vi "Interpolate Points_new.vi"(1 "End Point":cluster{"X":dbl, "Y":dbl}, 2 "Points number":dbl, 3 "Start Point":cluster{"X":dbl, "Y":dbl}) -> (0 "Output Point Array":cluster{"X":dbl, "Y":dbl}[](array[cluster]))   [LabVIEW 2013]
doc: "This VI interpolates at specified intervals between two points."
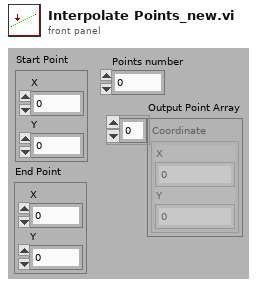
[diagram p1: front panel]
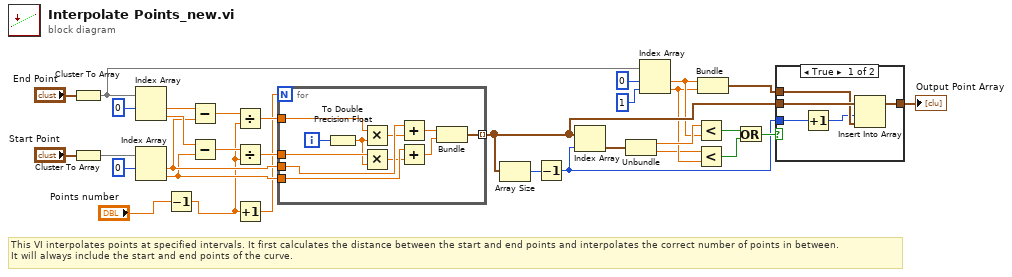
[diagram p0: block diagram]
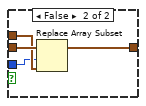
[diagram p2: hidden frame]
diagram:
  # "This VI interpolates points at specified intervals. It first calculates the distance between the start and end points and interpolates the correct number of points in between. \nIt will always include the start and end points of the curve."
  n1 = Cluster To Array(cluster="End Point") -> (array=w15:dbl[])
  n2 = Cluster To Array(cluster="Start Point") -> (array=w16:dbl[])
  n3 = Index Array(array=w15, index #1=0 ("index")) -> (element #1=w30:dbl, element #2=w27:dbl)  [unwired: 1 in]
  n4 = Index Array(array=w16, index #1=0 ("index")) -> (element #1=w26:dbl, element #2=w24:dbl)  [unwired: 1 in]
  n5 = Decrement(x="Points number") -> (x-1=w1:dbl)
  n6 = Subtract(x=w30, y=w26) -> (x-y=w29:dbl)
  n7 = Subtract(x=w27, y=w24) -> (x-y=w28:dbl)
  n8 = Divide(x=w29, y=w1) -> (x/y=w25:dbl)
  n9 = Divide(x=w28, y=w1) -> (x/y=w23:dbl)
  n10 = Increment(x=w1) -> (x+1=w22:dbl)
  n11 = for {
    N: w22 -> [_]
    tunnel: w26 -> [w43]
    tunnel: w25 -> [w42]
    tunnel: w24 -> [w40]
    tunnel: w23 -> [w39]
    tunnel: [w35] -> w9 mode=indexing
    i -> [w34]
    n12 = To Double Precision Float(number=w34) -> (double precision float=w33:dbl)
    n13 = Multiply(x=w42, y=w33) -> (x*y=w41:dbl)
    n14 = Multiply(x=w39, y=w33) -> (x*y=w38:dbl)
    n15 = Add(x=w43, y=w41) -> (x+y=w37:dbl)
    n16 = Add(x=w40, y=w38) -> (x+y=w36:dbl)
    n17 = Bundle(w37, w36) -> (w35:cluster{dbl, dbl})  [unwired: 1 out]
  }
  n18 = Array Size(array=w9) -> (size(s)=w18:i32)
  n19 = Decrement(x=w18) -> (x-1=w8:i32)
  n20 = Index Array(array=w9, index=w8) -> (element=w7:cluster{dbl, dbl})
  n21 = Unbundle(w7) -> (w6:dbl, w3:dbl)
  n22 = Index Array(array=w15, index #1=0 ("index"), index #2=1 ("index")) -> (element #1=w5:dbl, element #2=w4:dbl)
  n23 = Less?(x=w6, y=w5) -> (x < y?=w11:bool)
  n24 = Less?(x=w3, y=w4) -> (x < y?=w12:bool)
  n25 = Bundle("X"=w5, "X"=w4) -> (w19:cluster{"X":dbl, "X":dbl})  [unwired: 1 in]
  n26 = Or(x=w11, y=w12) -> (x .or. y?=w10:bool)
  n27 = case shown="True" w10 {
    tunnel: w9 -> [w48 w52]
    tunnel: w19 -> [w47 w51]
    tunnel: w8 -> [w45 w50]
    tunnel: [w46 w49] -> w13
    frame True {
      n28 = Increment(x=w45) -> (x+1=w44:i32)
      n29 = Insert Into Array(array=w48, index=w44, new element=w47) -> (w46:cluster{dbl, dbl}[])
    }
    frame False {
      n30 = Replace Array Subset(array=w52, new element=w51, index=w50) -> (w49:cluster{dbl, dbl}[])
    }
  }
  "Output Point Array" <- w13
